vi "Pack Data Element.vi"(6 "Data Elements":T1[](array[typedef]), 7 "Packed Offset In":i32, 9 "CIPC Offset In":i32, 10 "CIPC Data":u8[](array[numeric]), 11 "Packed Data In in":u8[](array[numeric])) -> (1 "CIPC Offset Out":i32, 3 "Packed Data In out":u8[](array[numeric]), 5 "Packed Offset Out":i32)   [LabVIEW 2021, in "CIF_NI_CIPC.lvlib"]
doc: "Packed data takes less space for transfer and for data logging. This will pack one CIPC data element. If the data element is part of an array this will need to be called multiple times to pack all the elements of the array."
uses:
  CIF_NI_CIPC.lvlib
  <vilib>/Utility/Data Type/Type Definitions/Data Type.ctl
  <vilib>/Utility/Data Type/NI_Data Type.lvlib
  TypeDefs/Data Element.ctl
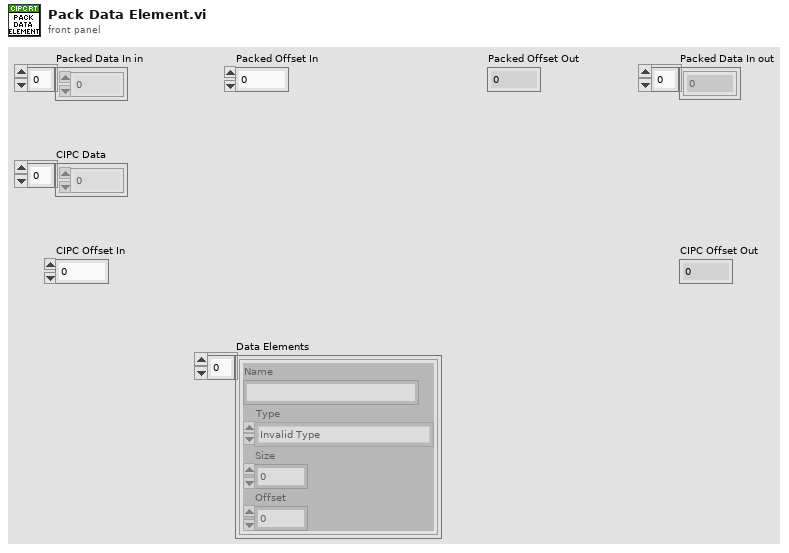
[diagram p1: front panel]
types:
  T1 = typedef "CIF_NI_CIPC.lvlib/Data Element.ctl" = cluster{"Name":string, "Type":T2, "Size":u32, "Offset":u32}
  T2 = typedef "NI_Data Type.lvlib/Data Type.ctl" = enum8{"Invalid Type", "Void", "I8", "I16", "I32", "I64", "U8", "U16", "U32", "U64", "Single Float", "Double Float", "Extended Float", "Single Complex", "Double Complex", "Extended Complex", "Enum U8", "Enum U16", "Enum U32", "Enum U64", "Single Float With Unit", "Double Float With Unit", "Extended Float With Unit", "Single Complex with Unit", "Double Complex with Unit", "Extended Complex with Unit", "Boolean", "String", "Path", "Picture", "Tag", "Array", "Cluster", "Variant", "LV Variant", "Waveform", "Timestamp", "Digital Waveform", "Digital Data", "ExpressData", "Refnum", "External Data", "VI", "Poly VI", "LabVIEW Class Instance", "Fixed Point", "Set Collection", "Map Collection"}
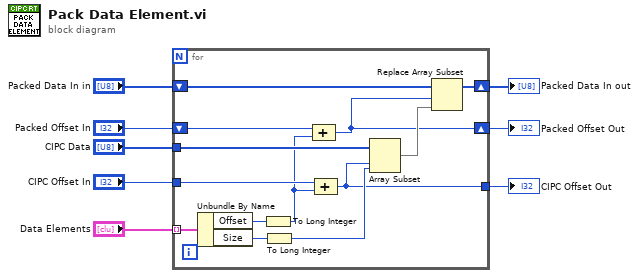
[diagram p0: block diagram]
diagram:
  n1 = for {
    tunnel: "Data Elements" -> [w21] mode=indexing
    shift-right: [w11] -> w8
    shift-left: "Packed Data In in" -> [w13]
    tunnel: "CIPC Offset In" -> [w17]
    shift-right: [w10] -> w2
    shift-left: "Packed Offset In" -> [w14]
    tunnel: "CIPC Data" -> [w18]
    tunnel: [w9] -> w1
    n2 = Unbundle By Name(w21) -> ("Offset"=w19:u32, "Size"=w20:u32)
    n3 = To Long Integer(number=w19) -> (32bit integer=w15:i32)
    n4 = To Long Integer(number=w20) -> (32bit integer=w16:i32)
    n5 = Compound Arithmetic op=ADD(w14, w15) -> (w10:i32)
    n6 = Compound Arithmetic op=ADD(w17, w15) -> (w9:i32)
    n7 = Array Subset(array=w18, index=w9, length=w16) -> (w12:u8[])
    n8 = Replace Array Subset(array=w13, new element=w12, index=w10) -> (w11:u8[])
  }
  "Packed Data In out" <- w8
  "Packed Offset Out" <- w2
  "CIPC Offset Out" <- w1
